vi "test_connection_ARM.vi"(8 "error in (no error)":errorcluster caption="エラー入力（エラーなし）", 11 "VISAリソース名":refnum<visa-resource-name>) -> (0 "error out":errorcluster caption="エラー出力", 2 "connected?":bool, 3 "VISAリソース名（出力）":refnum<visa-resource-name>)   [LabVIEW 2017]
uses:
  <vilib>/Instr/_visa.llb/VISA Configure Serial Port (Instr).vi
panel:
  out "レスポンス":string
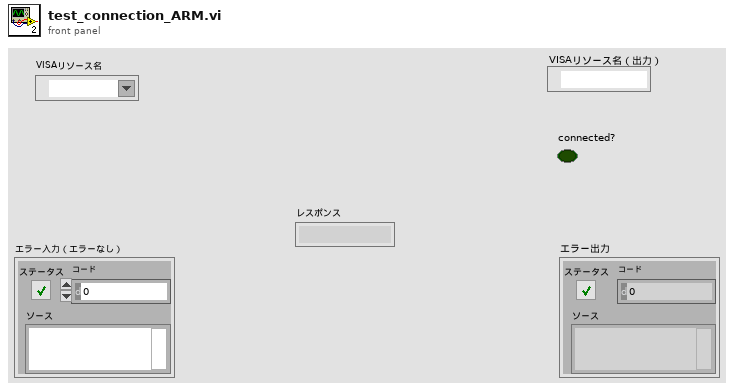
[diagram p1: front panel]
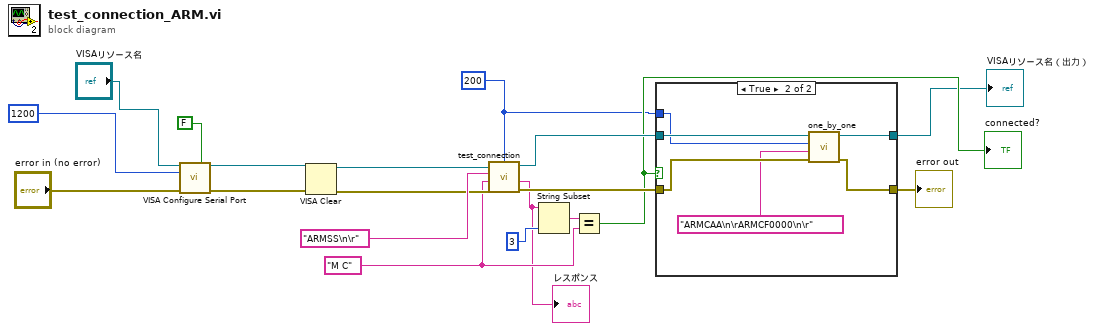
[diagram p0: block diagram]
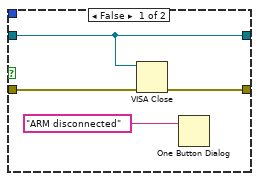
[diagram p2: hidden frame]
diagram:
  w1 = 200
  w5 = "M C" ("想定レスポンス")
  n1 = call-poly "VISA Configure Serial Port"("VISA resource name"="VISAリソース名", "Enable Termination\nChar (T)"=FALSE, "baud rate (9600)"=1200, "error in (no error)"="error in (no error)") -> ("VISA resource name out"=w11:refnum<visa-resource-name>, "error out"=w10:errorcluster)  [unwired: 10 in]
  n2 = VISA Clear(VISA resource name=w11, error in (no error)=w10) -> (VISA resource name out=w16:refnum<visa-resource-name>, error out=w15:errorcluster)
  n3 = call "test_connection.vi"("文字送信間隔 (500 ms)"=w1, "error in (no error)"=w15, "想定レスポンス"=w5, "コマンド"="ARMSS\n\r", "VISAリソース名"=w16) -> ("error out"=w18:errorcluster, "レスポンス"=w3:string, "VISAリソース名 （出力）"=w17:refnum<visa-resource-name>)  [unwired: 3 in, 1 out]
  "レスポンス" <- w3
  n4 = String Subset(string=w3, length (rest)=3) -> (substring=w6:string)  [unwired: 1 in]
  n5 = Equal?(x=w6, y=w5) -> (x = y?=w4:bool)
  "connected?" <- w4
  n6 = case shown="TRUE" w4 {
    tunnel: w18 -> [w23 w28]
    tunnel: w17 -> [w20 w29]
    tunnel: [w21 w26] -> w14
    tunnel: [w20 w25] -> w2
    tunnel: w1 -> [_ w24]
    frame False {
      n7 = VISA Close(VISA resource name=w20, error in (no error)=w23) -> (error out=w21:errorcluster)
      n8 = One Button Dialog(message="ARM disconnected") -> ()  [unwired: 1 in, 1 out]
    }
    frame True {
      n9 = call "one_by_one.vi"("error in (no error)"=w28, "入力文字"="ARMCAA\n\rARMCF0000\n\r", "待機 (200ms)"=w24, "VISAリソース名"=w29) -> ("error out"=w26:errorcluster, "VISAリソース名出力"=w25:refnum<visa-resource-name>)  [unwired: 6 in]
    }
  }
  "error out" <- w14
  "VISAリソース名（出力）" <- w2
